vi "FP Post Build.vi"() -> ()   [LabVIEW 2016]
uses:
  <userlib>/LevyLab/Build Support/PostBuildSupport/PostBuildSupport.lvclass
panel:
  in  "Package Version":string="4.50.1"
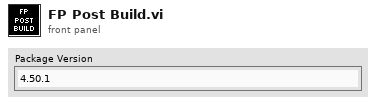
[diagram p1: front panel]
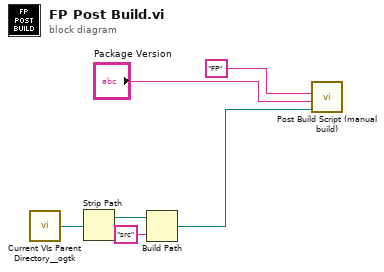
[diagram p0: block diagram]
diagram:
  n1 = call <userlib>:"Current VIs Parent Directory__ogtk.vi"() -> ("Parent Directory (+ Relative)"=w6:path)  [unwired: 5 in]
  n2 = Strip Path(path=w6) -> (stripped path=w5:path)  [unwired: 1 out]
  n3 = Build Path(base path=w5, name or relative path="src") -> (appended path=w1:path)
  n4 = call <userlib>:"Post Build Script (manual build).vi"("Package Source Folder"=w1, "Package Version"="Package Version", "Product Name"="FP") -> ()  [unwired: 8 in, 1 out]
